vi "GetOutputRelativePath.vi"(8 "error in (no error)":errorcluster, 11 "Path":path) -> (0 "error out":errorcluster, 3 "Output relative path":string)   [LabVIEW 2017]
uses:
  PathConfiguration.vi
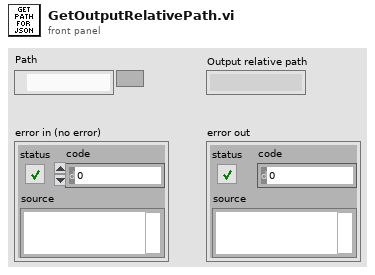
[diagram p1: front panel]
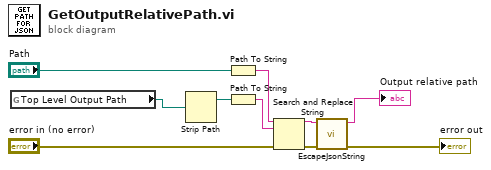
[diagram p0: block diagram]
diagram:
  n1 = global read "PathConfiguration.vi" "Top Level Output Path"() -> (w2:path)
  n2 = Strip Path(path=w2) -> (stripped path=w1:path)  [unwired: 1 out]
  n3 = Path To String(path="Path") -> (string=w9:string)
  n4 = Path To String(path=w1) -> (string=w3:string)
  n5 = Search and Replace String(input string=w9, search string=w3, error in="error in (no error)") -> (result string=w5:string, error out=w8:errorcluster)  [unwired: 5 in, 2 out]
  n6 = call "EscapeJsonString.vi"("error in (no error)"=w8, "String in"=w5) -> ("error out"=→"error out":errorcluster, "String out"=→"Output relative path":string)  [unwired: 8 in]
